vi "MAP.vi"() -> ()   [LabVIEW 2016]
panel:
  in  "Previous Button":bool
  out "Zvezda  2":picture
  out "Zarya  2":picture
  out "Solar panels  2":picture
  out "Soyuz  2":picture
  out "Radiators  2":picture
  out "Progress Supply Ship  2":picture
  out "Mobile Servicing Station  2":picture
  out "Kibo  2":picture
  out "Harmony  2":picture
  out "Destiny 2":picture
  out "Columbus  2":picture
  out "2D Picture":picture
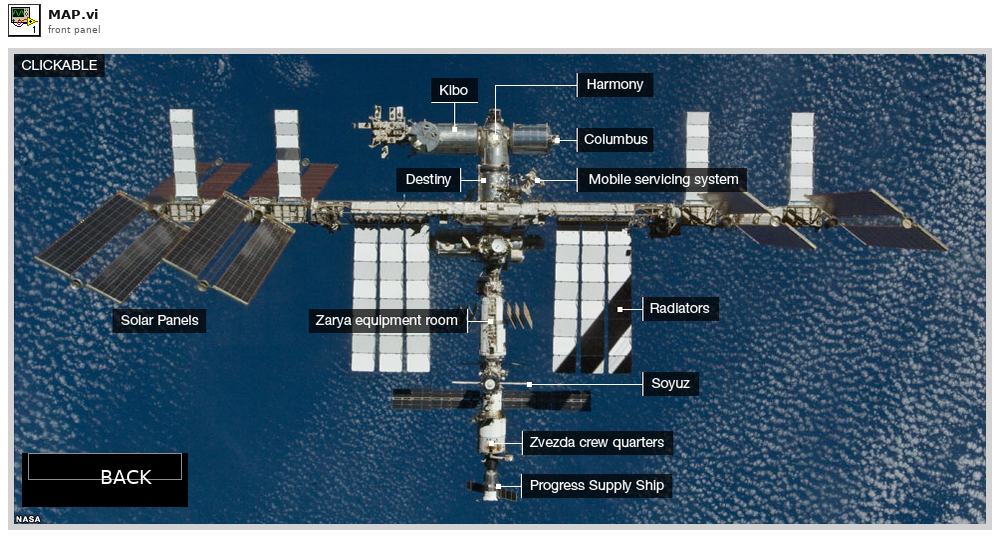
[diagram p1: front panel]
types:
  T1 = typedef "LVMouseTypeDef.ctl" = cluster{"Mouse Position":cluster{"X":i32, "Y":i32}, "Mouse Modifiers":cluster{"Button Down":bool, "Shift Mod":bool, "Menu Mod":bool, "Option Mod":bool}}
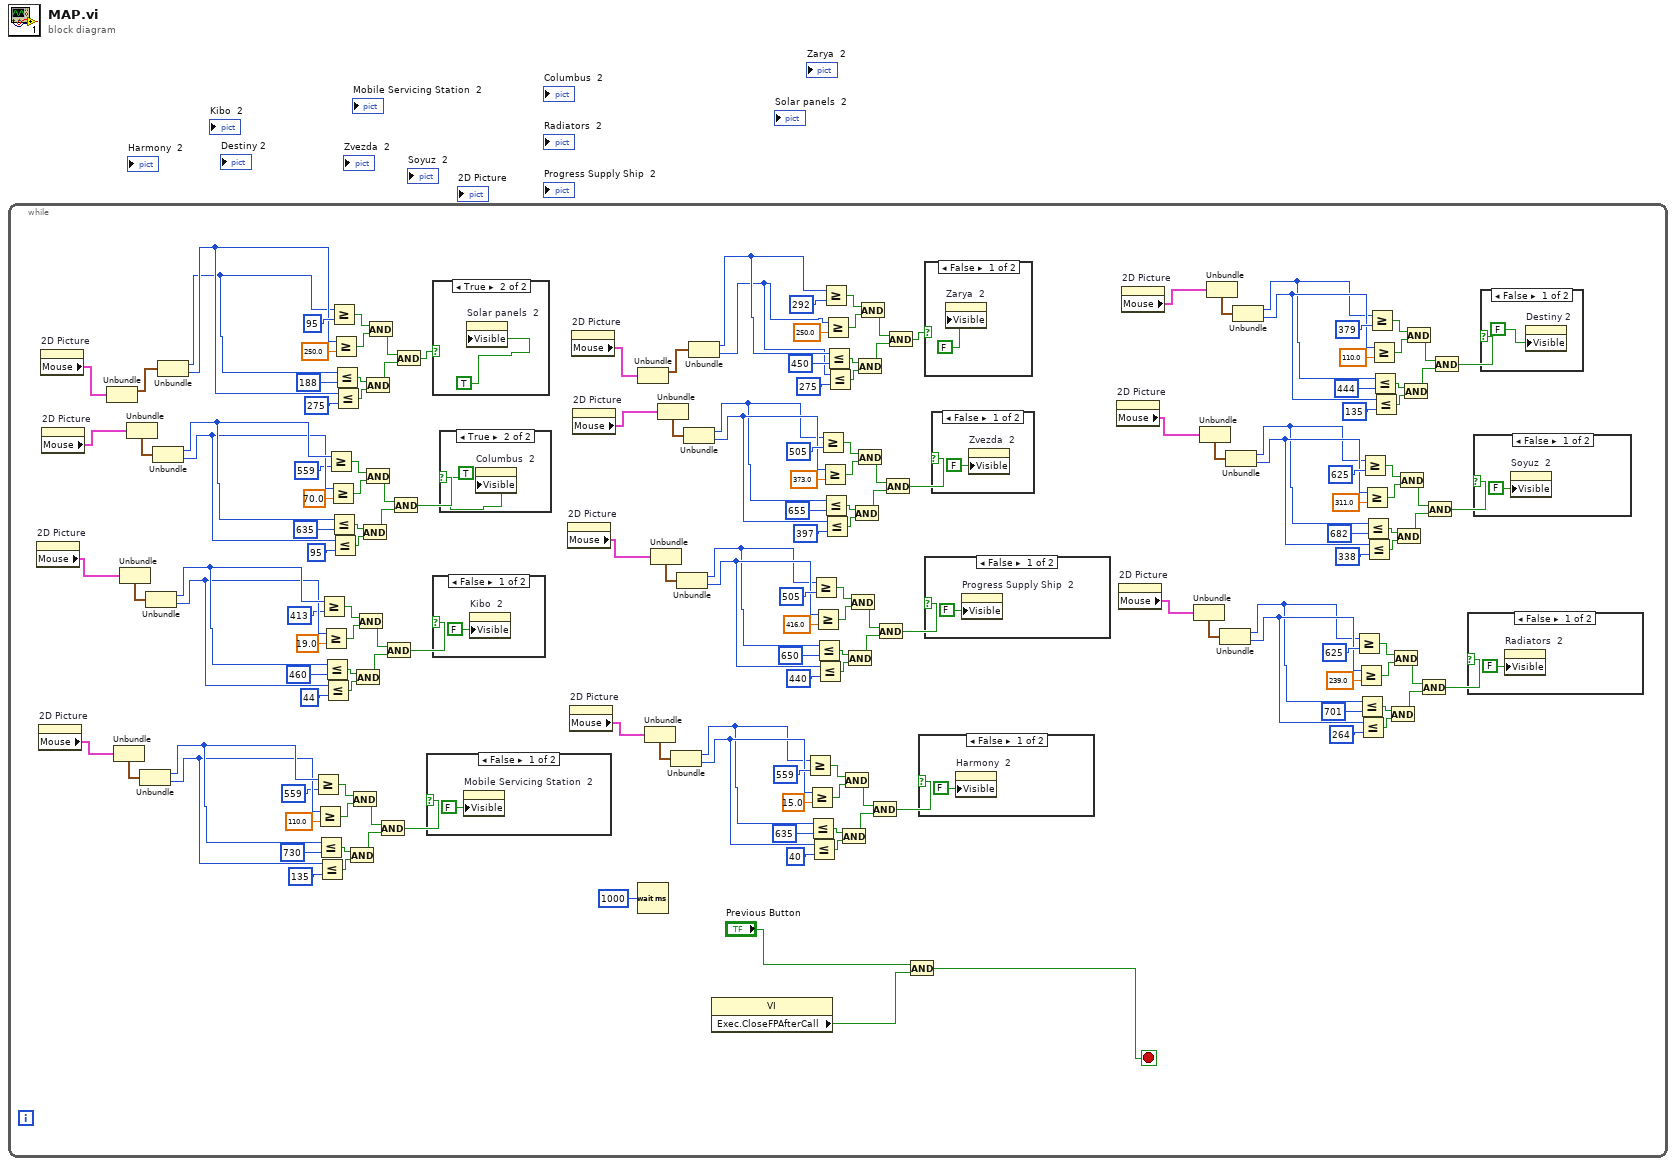
[diagram p0: block diagram]
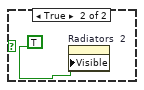
[diagram p2: hidden frame]
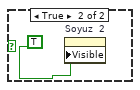
[diagram p3: hidden frame]
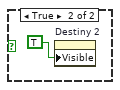
[diagram p4: hidden frame]
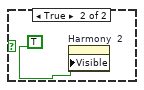
[diagram p5: hidden frame]
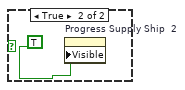
[diagram p6: hidden frame]
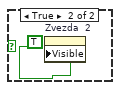
[diagram p7: hidden frame]
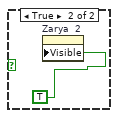
[diagram p8: hidden frame]
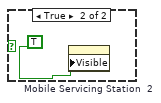
[diagram p9: hidden frame]
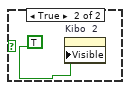
[diagram p10: hidden frame]
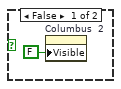
[diagram p11: hidden frame]
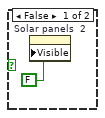
[diagram p12: hidden frame]
diagram:
  n1 = while {
    stop <- w1 stop-if-true
    n2 = property on="2D Picture" class="Pict"() -> ("Mouse"=w124:T1)  [unwired: 2 in, 2 out]
    n3 = property on="2D Picture" class="Pict"() -> ("Mouse"=w109:T1)  [unwired: 2 in, 2 out]
    n4 = property on="2D Picture" class="Pict"() -> ("Mouse"=w168:T1)  [unwired: 2 in, 2 out]
    n5 = property on="2D Picture" class="Pict"() -> ("Mouse"=w140:T1)  [unwired: 2 in, 2 out]
    n6 = Unbundle(w168) -> ("Mouse Position"=w167:cluster{"X":i32, "Y":i32})  [unwired: 1 out]
    n7 = Unbundle(w109) -> ("Mouse Position"=w110:cluster{"X":i32, "Y":i32})  [unwired: 1 out]
    n8 = Unbundle(w124) -> ("Mouse Position"=w125:cluster{"X":i32, "Y":i32})  [unwired: 1 out]
    n9 = Unbundle(w140) -> ("Mouse Position"=w141:cluster{"X":i32, "Y":i32})  [unwired: 1 out]
    n10 = Unbundle(w110) -> ("X"=w114:i32, "Y"=w113:i32)
    n11 = Unbundle(w125) -> ("X"=w129:i32, "Y"=w128:i32)
    n12 = Unbundle(w141) -> ("X"=w145:i32, "Y"=w144:i32)
    n13 = Unbundle(w167) -> ("X"=w163:i32, "Y"=w164:i32)
    n14 = Greater Or Equal?(x=w114, y=559) -> (x >= y?=w119:bool)
    n15 = Greater Or Equal?(x=w113, y=110.0) -> (x >= y?=w120:bool)
    n16 = Less Or Equal?(x=w114, y=730) -> (x <= y?=w117:bool)
    n17 = Less Or Equal?(x=w113, y=135) -> (x <= y?=w118:bool)
    n18 = Greater Or Equal?(x=w129, y=413) -> (x >= y?=w134:bool)
    n19 = Greater Or Equal?(x=w128, y=19.0) -> (x >= y?=w135:bool)
    n20 = Less Or Equal?(x=w129, y=460) -> (x <= y?=w132:bool)
    n21 = Less Or Equal?(x=w128, y=44) -> (x <= y?=w133:bool)
    n22 = Greater Or Equal?(x=w145, y=559) -> (x >= y?=w150:bool)
    n23 = Greater Or Equal?(x=w144, y=70.0) -> (x >= y?=w151:bool)
    n24 = Greater Or Equal?(x=w163, y=95) -> (x >= y?=w158:bool)
    n25 = Less Or Equal?(x=w145, y=635) -> (x <= y?=w148:bool)
    n26 = Less Or Equal?(x=w144, y=95) -> (x <= y?=w149:bool)
    n27 = Greater Or Equal?(x=w164, y=250.0) -> (x >= y?=w157:bool)
    n28 = Less Or Equal?(x=w163, y=188) -> (x <= y?=w160:bool)
    n29 = Less Or Equal?(x=w164, y=275) -> (x <= y?=w159:bool)
    n30 = And(x=w117, y=w118) -> (x .and. y?=w122:bool)
    n31 = And(x=w119, y=w120) -> (x .and. y?=w121:bool)
    n32 = And(x=w132, y=w133) -> (x .and. y?=w137:bool)
    n33 = And(x=w134, y=w135) -> (x .and. y?=w136:bool)
    n34 = And(x=w148, y=w149) -> (x .and. y?=w153:bool)
    n35 = And(x=w160, y=w159) -> (x .and. y?=w155:bool)
    n36 = And(x=w150, y=w151) -> (x .and. y?=w152:bool)
    n37 = And(x=w158, y=w157) -> (x .and. y?=w156:bool)
    n38 = And(x=w121, y=w122) -> (x .and. y?=w123:bool)
    n39 = And(x=w136, y=w137) -> (x .and. y?=w138:bool)
    n40 = And(x=w152, y=w153) -> (x .and. y?=w154:bool)
    n41 = And(x=w156, y=w155) -> (x .and. y?=w139:bool)
    n42 = case shown="False" w123 {
      frame False {
        n43 = property on="Mobile Servicing Station  2" class="Pict"("Visible"=FALSE) -> ()  [unwired: 2 in, 2 out]
      }
      frame True {
        n44 = property on="Mobile Servicing Station  2" class="Pict"("Visible"=TRUE) -> ()  [unwired: 2 in, 2 out]
      }
    }
    n45 = case shown="True" w139 {
      frame False {
        n46 = property on="Solar panels  2" class="Pict"("Visible"=FALSE) -> ()  [unwired: 2 in, 2 out]
      }
      frame True {
        n47 = property on="Solar panels  2" class="Pict"("Visible"=TRUE) -> ()  [unwired: 2 in, 2 out]
      }
    }
    n48 = case shown="False" w138 {
      frame False {
        n49 = property on="Kibo  2" class="Pict"("Visible"=FALSE) -> ()  [unwired: 2 in, 2 out]
      }
      frame True {
        n50 = property on="Kibo  2" class="Pict"("Visible"=TRUE) -> ()  [unwired: 2 in, 2 out]
      }
    }
    n51 = case shown="True" w154 {
      frame False {
        n52 = property on="Columbus  2" class="Pict"("Visible"=FALSE) -> ()  [unwired: 2 in, 2 out]
      }
      frame True {
        n53 = property on="Columbus  2" class="Pict"("Visible"=TRUE) -> ()  [unwired: 2 in, 2 out]
      }
    }
    n54 = property on="2D Picture" class="Pict"() -> ("Mouse"=w93:T1)  [unwired: 2 in, 2 out]
    n55 = property on="2D Picture" class="Pict"() -> ("Mouse"=w108:T1)  [unwired: 2 in, 2 out]
    n56 = property on="2D Picture" class="Pict"() -> ("Mouse"=w50:T1)  [unwired: 2 in, 2 out]
    n57 = property on="2D Picture" class="Pict"() -> ("Mouse"=w77:T1)  [unwired: 2 in, 2 out]
    n58 = Unbundle(w50) -> ("Mouse Position"=w51:cluster{"X":i32, "Y":i32})  [unwired: 1 out]
    n59 = Wait (ms)(milliseconds to wait=u32 1000) -> ()  [unwired: 1 out]
    n60 = Unbundle(w108) -> ("Mouse Position"=w107:cluster{"X":i32, "Y":i32})  [unwired: 1 out]
    n61 = Unbundle(w93) -> ("Mouse Position"=w92:cluster{"X":i32, "Y":i32})  [unwired: 1 out]
    n62 = Unbundle(w77) -> ("Mouse Position"=w76:cluster{"X":i32, "Y":i32})  [unwired: 1 out]
    n63 = Unbundle(w107) -> ("X"=w103:i32, "Y"=w104:i32)
    n64 = Unbundle(w92) -> ("X"=w88:i32, "Y"=w89:i32)
    n65 = Unbundle(w76) -> ("X"=w72:i32, "Y"=w73:i32)
    n66 = Unbundle(w51) -> ("X"=w54:i32, "Y"=w49:i32)
    n67 = property class="VI"() -> ("Exec.CloseFPAfterCall"=w2:bool)  [unwired: 2 in, 2 out]
    n68 = Greater Or Equal?(x=w103, y=559) -> (x >= y?=w98:bool)
    n69 = Greater Or Equal?(x=w104, y=15.0) -> (x >= y?=w97:bool)
    n70 = Less Or Equal?(x=w103, y=635) -> (x <= y?=w100:bool)
    n71 = Less Or Equal?(x=w104, y=40) -> (x <= y?=w99:bool)
    n72 = Greater Or Equal?(x=w88, y=505) -> (x >= y?=w83:bool)
    n73 = Greater Or Equal?(x=w89, y=416.0) -> (x >= y?=w82:bool)
    n74 = Less Or Equal?(x=w88, y=650) -> (x <= y?=w85:bool)
    n75 = Less Or Equal?(x=w89, y=440) -> (x <= y?=w84:bool)
    n76 = Greater Or Equal?(x=w72, y=505) -> (x >= y?=w67:bool)
    n77 = Greater Or Equal?(x=w73, y=373.0) -> (x >= y?=w66:bool)
    n78 = Greater Or Equal?(x=w54, y=292) -> (x >= y?=w59:bool)
    n79 = Less Or Equal?(x=w72, y=655) -> (x <= y?=w69:bool)
    n80 = Less Or Equal?(x=w73, y=397) -> (x <= y?=w68:bool)
    n81 = Greater Or Equal?(x=w49, y=250.0) -> (x >= y?=w60:bool)
    n82 = Less Or Equal?(x=w54, y=450) -> (x <= y?=w57:bool)
    n83 = Less Or Equal?(x=w49, y=275) -> (x <= y?=w58:bool)
    n84 = And(x=w100, y=w99) -> (x .and. y?=w95:bool)
    n85 = And(x=w98, y=w97) -> (x .and. y?=w96:bool)
    n86 = And(x=w85, y=w84) -> (x .and. y?=w80:bool)
    n87 = And(x=w83, y=w82) -> (x .and. y?=w81:bool)
    n88 = And(x=w69, y=w68) -> (x .and. y?=w64:bool)
    n89 = And(x=w57, y=w58) -> (x .and. y?=w62:bool)
    n90 = And(x=w67, y=w66) -> (x .and. y?=w65:bool)
    n91 = And(x=w59, y=w60) -> (x .and. y?=w61:bool)
    n92 = And(x=w96, y=w95) -> (x .and. y?=w94:bool)
    n93 = And(x=w81, y=w80) -> (x .and. y?=w79:bool)
    n94 = And(x=w65, y=w64) -> (x .and. y?=w63:bool)
    n95 = And(x=w61, y=w62) -> (x .and. y?=w78:bool)
    n96 = And(x="Previous Button", y=w2) -> (x .and. y?=w1:bool)
    n97 = case shown="False" w94 {
      frame False {
        n98 = property on="Harmony  2" class="Pict"("Visible"=FALSE) -> ()  [unwired: 2 in, 2 out]
      }
      frame True {
        n99 = property on="Harmony  2" class="Pict"("Visible"=TRUE) -> ()  [unwired: 2 in, 2 out]
      }
    }
    n100 = case shown="False" w78 {
      frame False {
        n101 = property on="Zarya  2" class="Pict"("Visible"=FALSE) -> ()  [unwired: 2 in, 2 out]
      }
      frame True {
        n102 = property on="Zarya  2" class="Pict"("Visible"=TRUE) -> ()  [unwired: 2 in, 2 out]
      }
    }
    n103 = case shown="False" w79 {
      frame False {
        n104 = property on="Progress Supply Ship  2" class="Pict"("Visible"=FALSE) -> ()  [unwired: 2 in, 2 out]
      }
      frame True {
        n105 = property on="Progress Supply Ship  2" class="Pict"("Visible"=TRUE) -> ()  [unwired: 2 in, 2 out]
      }
    }
    n106 = case shown="False" w63 {
      frame False {
        n107 = property on="Zvezda  2" class="Pict"("Visible"=FALSE) -> ()  [unwired: 2 in, 2 out]
      }
      frame True {
        n108 = property on="Zvezda  2" class="Pict"("Visible"=TRUE) -> ()  [unwired: 2 in, 2 out]
      }
    }
    n109 = property on="2D Picture" class="Pict"() -> ("Mouse"=w33:T1)  [unwired: 2 in, 2 out]
    n110 = property on="2D Picture" class="Pict"() -> ("Mouse"=w48:T1)  [unwired: 2 in, 2 out]
    n111 = property on="2D Picture" class="Pict"() -> ("Mouse"=w18:T1)  [unwired: 2 in, 2 out]
    n112 = Unbundle(w48) -> ("Mouse Position"=w47:cluster{"X":i32, "Y":i32})  [unwired: 1 out]
    n113 = Unbundle(w33) -> ("Mouse Position"=w32:cluster{"X":i32, "Y":i32})  [unwired: 1 out]
    n114 = Unbundle(w18) -> ("Mouse Position"=w17:cluster{"X":i32, "Y":i32})  [unwired: 1 out]
    n115 = Unbundle(w47) -> ("X"=w43:i32, "Y"=w44:i32)
    n116 = Unbundle(w32) -> ("X"=w28:i32, "Y"=w29:i32)
    n117 = Unbundle(w17) -> ("X"=w13:i32, "Y"=w14:i32)
    n118 = Greater Or Equal?(x=w43, y=625) -> (x >= y?=w38:bool)
    n119 = Greater Or Equal?(x=w44, y=239.0) -> (x >= y?=w37:bool)
    n120 = Less Or Equal?(x=w43, y=701) -> (x <= y?=w40:bool)
    n121 = Less Or Equal?(x=w44, y=264) -> (x <= y?=w39:bool)
    n122 = Greater Or Equal?(x=w28, y=625) -> (x >= y?=w23:bool)
    n123 = Greater Or Equal?(x=w29, y=311.0) -> (x >= y?=w22:bool)
    n124 = Less Or Equal?(x=w28, y=682) -> (x <= y?=w25:bool)
    n125 = Less Or Equal?(x=w29, y=338) -> (x <= y?=w24:bool)
    n126 = Greater Or Equal?(x=w13, y=379) -> (x >= y?=w8:bool)
    n127 = Greater Or Equal?(x=w14, y=110.0) -> (x >= y?=w7:bool)
    n128 = Less Or Equal?(x=w13, y=444) -> (x <= y?=w10:bool)
    n129 = Less Or Equal?(x=w14, y=135) -> (x <= y?=w9:bool)
    n130 = And(x=w40, y=w39) -> (x .and. y?=w35:bool)
    n131 = And(x=w38, y=w37) -> (x .and. y?=w36:bool)
    n132 = And(x=w25, y=w24) -> (x .and. y?=w20:bool)
    n133 = And(x=w23, y=w22) -> (x .and. y?=w21:bool)
    n134 = And(x=w10, y=w9) -> (x .and. y?=w5:bool)
    n135 = And(x=w8, y=w7) -> (x .and. y?=w6:bool)
    n136 = And(x=w36, y=w35) -> (x .and. y?=w34:bool)
    n137 = And(x=w21, y=w20) -> (x .and. y?=w19:bool)
    n138 = And(x=w6, y=w5) -> (x .and. y?=w4:bool)
    n139 = case shown="False" w34 {
      frame False {
        n140 = property on="Radiators  2" class="Pict"("Visible"=FALSE) -> ()  [unwired: 2 in, 2 out]
      }
      frame True {
        n141 = property on="Radiators  2" class="Pict"("Visible"=TRUE) -> ()  [unwired: 2 in, 2 out]
      }
    }
    n142 = case shown="False" w19 {
      frame False {
        n143 = property on="Soyuz  2" class="Pict"("Visible"=FALSE) -> ()  [unwired: 2 in, 2 out]
      }
      frame True {
        n144 = property on="Soyuz  2" class="Pict"("Visible"=TRUE) -> ()  [unwired: 2 in, 2 out]
      }
    }
    n145 = case shown="False" w4 {
      frame False {
        n146 = property on="Destiny 2" class="Pict"("Visible"=FALSE) -> ()  [unwired: 2 in, 2 out]
      }
      frame True {
        n147 = property on="Destiny 2" class="Pict"("Visible"=TRUE) -> ()  [unwired: 2 in, 2 out]
      }
    }
  }
